vi "Wait Until Text Out.vi"(1 "Wait Until Ctr":T2={"Available Data"=[], "Target Value"=0.0, "Condition"=enum."= target value", "xxx%"=0.0, "Timeout (sec)"=30000.0, "selected index"=0, "initial wait (sec)"=0.0}) -> (0 "Command text":string[][](array[string]))   [LabVIEW 2019]
uses:
  Wait Until.ctl
  Wait Until condition.ctl
panel:
  out "Wait Until Condition":T1=enum."= target value"
  out "String Cluster":T3
  # "Wait Until Command"
  # "This command waits until 'DATA' value in NML Data Acquisition program meets user specified the condition."
  # "Select DATA to monitor"
  # "Enter Target value"
  # "Specifiy 'wait until' condition"
  # "Wait until DATA  is"
  # "(Specify"
  # "if necessary)"
  # "Enter 'Time out' here"
  # "sec"
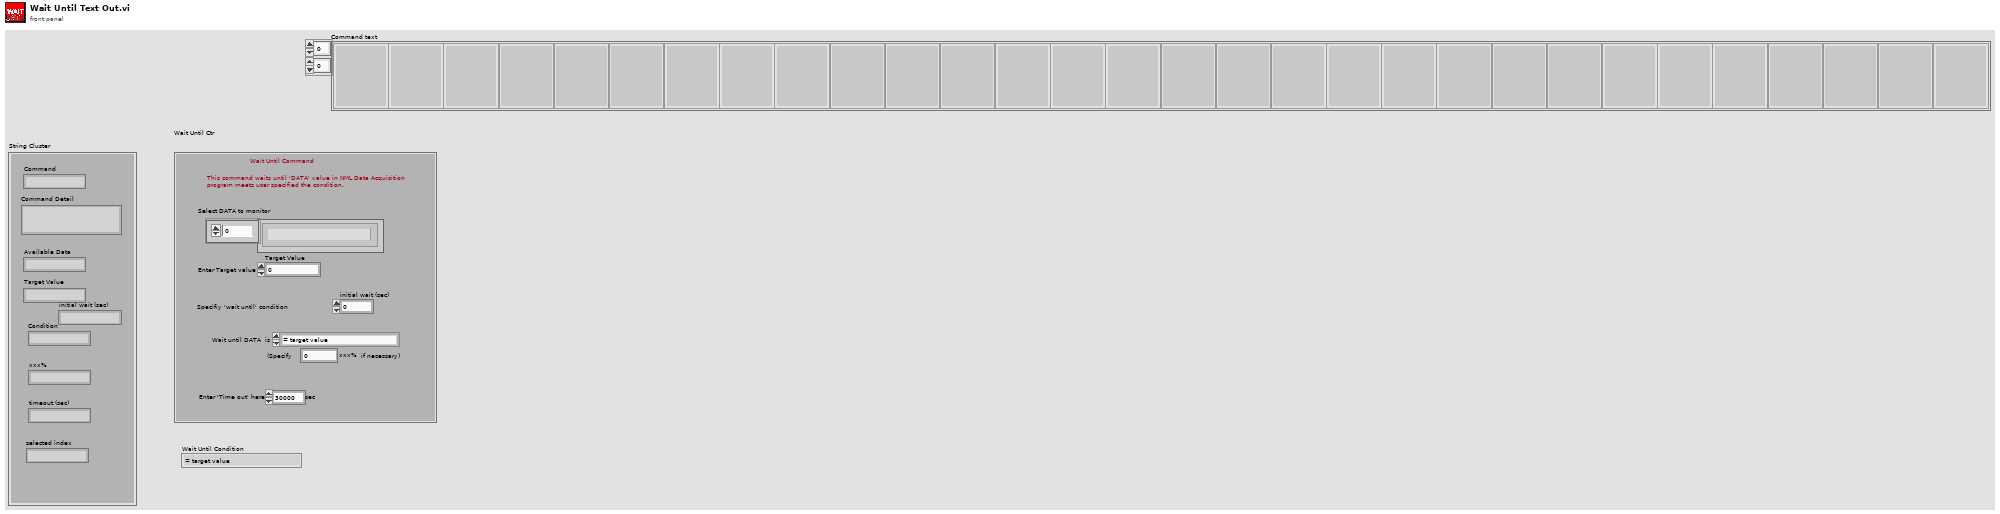
[diagram p1: front panel]
types:
  T1 = typedef "Wait Until condition.ctl" = enum16{"within xxx% of target value", "<= target value", ">= target value", "= target value"}
  T2 = typedef "Wait Until.ctl" = cluster{"Available Data":string[], "Target Value":dbl, "Condition":T1, "xxx%":dbl, "Timeout (sec)":dbl, "selected index":u32, "initial wait (sec)":dbl}
  T3 = cluster{"Command":string, "Command Detail":string, "Available Data":string, "Target Value":string, "Condition":string, "xxx%":string, "timeout (sec)":string, "selected index":string, "initial wait (sec)":string}
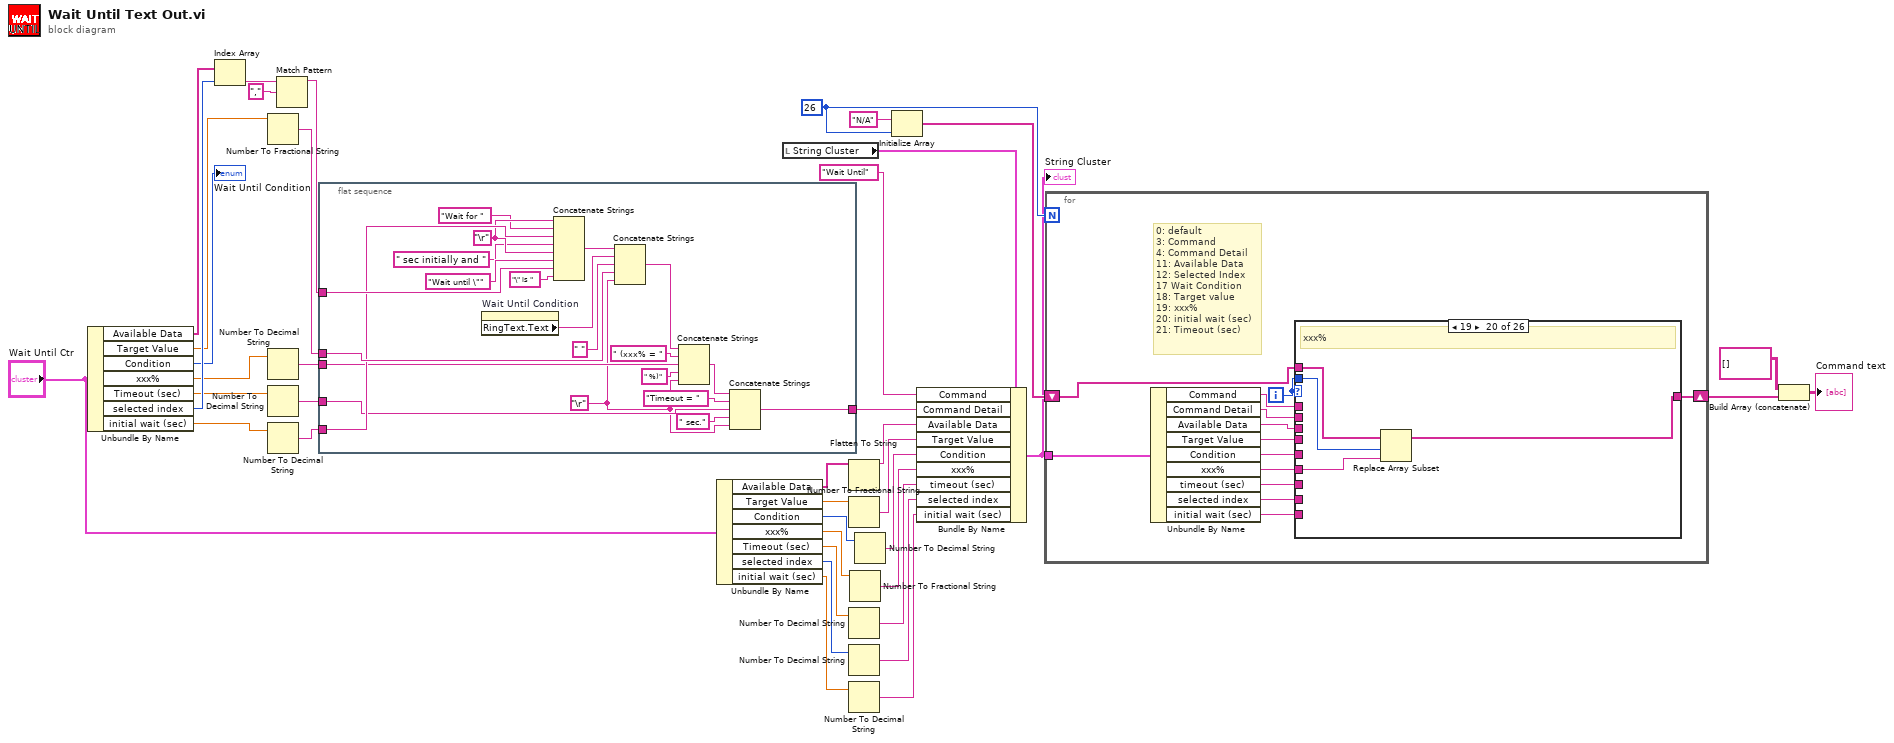
[diagram p0: block diagram]
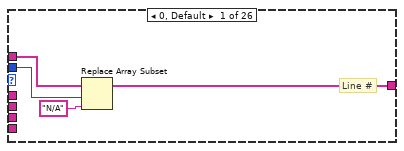
[diagram p2: hidden frame]
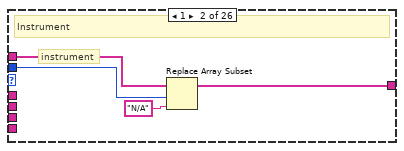
[diagram p3: hidden frame]
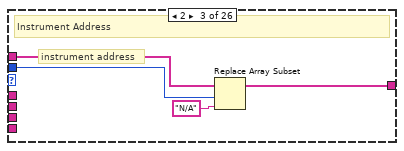
[diagram p4: hidden frame]
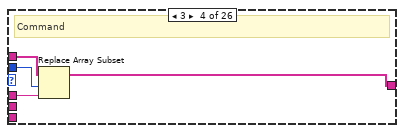
[diagram p5: hidden frame]
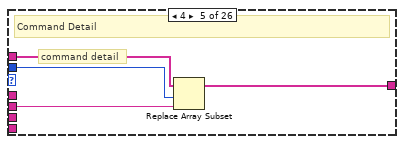
[diagram p6: hidden frame]
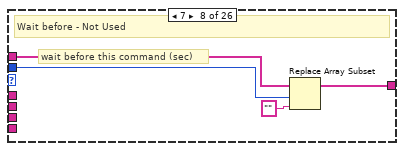
[diagram p9: hidden frame]
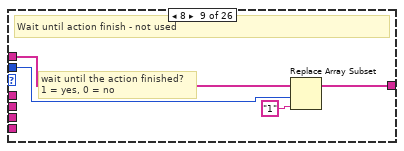
[diagram p10: hidden frame]
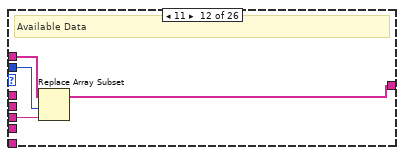
[diagram p13: hidden frame]
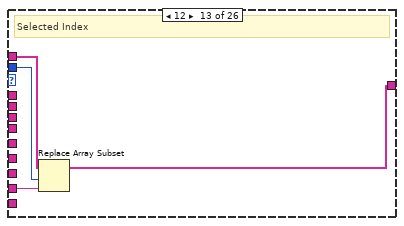
[diagram p14: hidden frame]
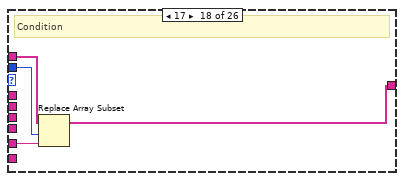
[diagram p19: hidden frame]
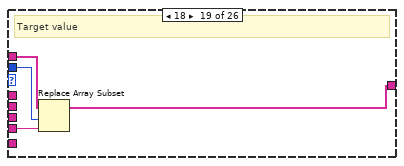
[diagram p20: hidden frame]
diagram:
  w14 = 26
  n1 = Unbundle By Name("Wait Until Ctr") -> ("Available Data"=w39:string[], "Target Value"=w34:dbl, "Condition"=→"Wait Until Condition":T1, "xxx%"=w4:dbl, "Timeout (sec)"=w2:dbl, "selected index"=w38:u32, "initial wait (sec)"=w6:dbl)
  n2 = Index Array(array=w39, index=w38) -> (element=w37:string)
  n3 = Number To Fractional String(number=w34) -> (F-format string=w33:string)  [unwired: 3 in]
  n4 = Number To Decimal String(number=w4) -> (decimal integer string=w3:string)  [unwired: 1 in]
  n5 = Number To Decimal String(number=w2) -> (decimal integer string=w1:string)  [unwired: 1 in]
  n6 = Number To Decimal String(number=w6) -> (decimal integer string=w5:string)  [unwired: 1 in]
  n7 = Match Pattern(string=w37, regular expression="," ("search string")) -> (before substring=w35:string)  [unwired: 1 in, 3 out]
  n8 = flat-sequence {
    tunnel: w35 -> [w59]
    tunnel: w33 -> [w55]
    tunnel: [w40] -> w30
    tunnel: w5 -> [w53]
    tunnel: w3 -> [w47]
    tunnel: w1 -> [w43]
    frame #0 {
      w41 = "\r"
      w52 = "\r"
      n9 = property on="Wait Until Condition" class="Enum (strict)"() -> ("RingText.Text"=w54:string)  [unwired: 2 in, 2 out]
      n10 = Concatenate Strings(w52, "Wait for " ("string"), w53, " sec initially and " ("string"), w52, "Wait until \"" ("string"), w59, "\" is " ("string")) -> (w57:string)
      n11 = Concatenate Strings(w57, w54, " " ("string"), w55, w41) -> (w49:string)
      n12 = Concatenate Strings(w49, " (xxx% = " ("string"), w47, " %)" ("string"), w41) -> (w45:string)
      n13 = Concatenate Strings(w45, "Timeout = " ("string"), w43, " sec." ("string"), w41) -> (w40:string)
    }
  }
  n14 = Unbundle By Name("Wait Until Ctr") -> ("Available Data"=w29:string[], "Target Value"=w27:dbl, "Condition"=w24:T1, "xxx%"=w22:dbl, "Timeout (sec)"=w20:dbl, "selected index"=w18:u32, "initial wait (sec)"=w8:dbl)
  n15 = local read "String Cluster"() -> (w16:T3)
  n16 = Flatten To String(anything=w29) -> (data string=w28:string)  [unwired: 3 in, 2 out]
  n17 = Number To Fractional String(number=w27) -> (F-format string=w26:string)  [unwired: 3 in]
  n18 = Number To Decimal String(number=w20) -> (decimal integer string=w19:string)  [unwired: 1 in]
  n19 = Number To Decimal String(number=w18) -> (decimal integer string=w17:string)  [unwired: 1 in]
  n20 = Number To Decimal String(number=w8) -> (decimal integer string=w7:string)  [unwired: 1 in]
  n21 = Number To Fractional String(number=w22) -> (F-format string=w21:string)  [unwired: 3 in]
  n22 = Number To Decimal String(number=w24) -> (decimal integer string=w23:string)  [unwired: 1 in]
  n23 = Initialize Array("N/A", w14) -> (w13:string[])
  n24 = Bundle By Name(cluster=w16, "Command"="Wait Until", "Command Detail"=w30, "Available Data"=w28, "Target Value"=w26, "Condition"=w23, "xxx%"=w21, "timeout (sec)"=w19, "selected index"=w17, "initial wait (sec)"=w7) -> (w12:T3)
  "String Cluster" <- w12
  n25 = for {
    N: w14 -> [_]
    shift-right: [w72] -> w10
    shift-left: w13 -> [w73]
    tunnel: w12 -> [w70]
    i -> [w71]
    # "0: default\n3: Command\n4: Command Detail\n11: Available Data\n12: Selected Index\n17 Wait Condition\n18: Target value\n19: xxx%\n20: initial wait (sec)\n21: Timeout (sec)"
    n26 = Unbundle By Name(w70) -> ("Command"=w69:string, "Command Detail"=w68:string, "Available Data"=w67:string, "Target Value"=w64:string, "Condition"=w65:string, "xxx%"=w63:string, "timeout (sec)"=w62:string, "selected index"=w66:string, "initial wait (sec)"=w61:string)
    n27 = case shown="19" w71 {
      tunnel: w71 -> [w76 w81 w85 w88 w92 _ _ w97 w101 _ _ w107 w111 _ _ _ _ w119 w123 w127 w131 w135 _ _ _ _]
      tunnel: w73 -> [w77 w80 w84 w89 w93 w94 w95 w99 w103 w104 w105 w108 w113 w114 w115 w116 w117 w121 w125 w129 w133 w137 w138 w139 w140 w141]
      tunnel: [w74 w79 w83 w87 w91 w94 w95 w98 w102 w104 w105 w109 w112 w114 w115 w116 w117 w120 w124 w128 w132 w136 w138 w139 w140 w141] -> w72
      tunnel: w69 -> [_ _ _ w86 _ _ _ _ _ _ _ _ _ _ _ _ _ _ _ _ _ _ _ _ _ _]
      tunnel: w68 -> [_ _ _ _ w90 _ _ _ _ _ _ _ _ _ _ _ _ _ _ _ _ _ _ _ _ _]
      tunnel: w67 -> [_ _ _ _ _ _ _ _ _ _ _ w106 _ _ _ _ _ _ _ _ _ _ _ _ _ _]
      tunnel: w66 -> [_ _ _ _ _ _ _ _ _ _ _ _ w110 _ _ _ _ _ _ _ _ _ _ _ _ _]
      tunnel: w65 -> [_ _ _ _ _ _ _ _ _ _ _ _ _ _ _ _ _ w118 _ _ _ _ _ _ _ _]
      tunnel: w64 -> [_ _ _ _ _ _ _ _ _ _ _ _ _ _ _ _ _ _ w122 _ _ _ _ _ _ _]
      tunnel: w63 -> [_ _ _ _ _ _ _ _ _ _ _ _ _ _ _ _ _ _ _ w126 _ _ _ _ _ _]
      tunnel: w62 -> [_ _ _ _ _ _ _ _ _ _ _ _ _ _ _ _ _ _ _ _ _ w134 _ _ _ _]
      tunnel: w61 -> [_ _ _ _ _ _ _ _ _ _ _ _ _ _ _ _ _ _ _ _ w130 _ _ _ _ _]
      frame 0, Default {
        # "Line #"
        n28 = Replace Array Subset(array=w77, new element="N/A", index=w76) -> (w74:string[])
      }
      frame 1 {
        # "instrument"
        # "Instrument"
        n29 = Replace Array Subset(array=w80, new element="N/A", index=w81) -> (w79:string[])
      }
      frame 2 {
        # "instrument address"
        # "Instrument Address"
        n30 = Replace Array Subset(array=w84, new element="N/A" ("new element/subarray"), index=w85) -> (w83:string[])
      }
      frame 3 {
        # "Command"
        n31 = Replace Array Subset(array=w89, new element=w86, index=w88) -> (w87:string[])
      }
      frame 4 {
        # "command detail"
        # "Command Detail"
        n32 = Replace Array Subset(array=w93, new element=w90, index=w92) -> (w91:string[])
      }
      frame 5 {
        # "in  case 1"
        # "Nothing"
      }
      frame 6 {
        # "in case 2"
        # "Nothing"
      }
      frame 7 {
        # "wait before this command (sec)"
        # "Wait before - Not Used"
        n33 = Replace Array Subset(array=w99, new element="" ("new element/subarray"), index=w97) -> (w98:string[])
      }
      frame 8 {
        # "wait until the action finished?\n1 = yes, 0 = no"
        # "Wait until action finish - not used"
        n34 = Replace Array Subset(array=w103, new element="1", index=w101) -> (w102:string[])
      }
      frame 9 {
        # "extra wait (sec)"
        # "Nothing"
      }
      frame 10 {
        # "Nothing"
      }
      frame 11 {
        # "Available Data"
        n35 = Replace Array Subset(array=w108, new element=w106, index=w107) -> (w109:string[])
      }
      frame 12 {
        # "Selected Index"
        n36 = Replace Array Subset(array=w113, new element=w110, index=w111) -> (w112:string[])
      }
      frame 13 {
        # "Nothing"
      }
      frame 14 {
        # "Nothing"
      }
      frame 15 {
        # "Nothing"
      }
      frame 16 {
        # "Nothing"
      }
      frame 17 {
        # "Condition"
        n37 = Replace Array Subset(array=w121, new element=w118, index=w119) -> (w120:string[])
      }
      frame 18 {
        # "Target value"
        n38 = Replace Array Subset(array=w125, new element=w122, index=w123) -> (w124:string[])
      }
      frame 19 {
        # "xxx%"
        n39 = Replace Array Subset(array=w129, new element=w126, index=w127) -> (w128:string[])
      }
      frame 20 {
        # "initial wait (sec)"
        n40 = Replace Array Subset(array=w133, new element=w130, index=w131) -> (w132:string[])
      }
      frame 21 {
        # "Timeout (sec)"
        n41 = Replace Array Subset(array=w137, new element=w134, index=w135) -> (w136:string[])
      }
      frame 22 {
      }
      frame 23 {
      }
      frame 24 {
      }
      frame 25 {
      }
    }
  }
  n42 = Build Array (concatenate)(string[][] [], w10) -> (→"Command text":string[][])
